vi "visualizrion.vi"() -> ()   [LabVIEW 2024]
uses:
  <vilib>/picture/3D Picture Control/Object/Create Object (name).vi
  <vilib>/Utility/file.llb/Read Delimited Spreadsheet (string).vi
  <vilib>/picture/3D Picture Control/Helpers/Set Light (no reference).vi
  <vilib>/picture/3D Picture Control/NI_3D Picture Control.lvlib
panel:
  out "Slide":u8(slide) scale=0.0..100.0
  in  "stop":bool
  out "3D Picture 2":refnum<vi>(3d-picture)
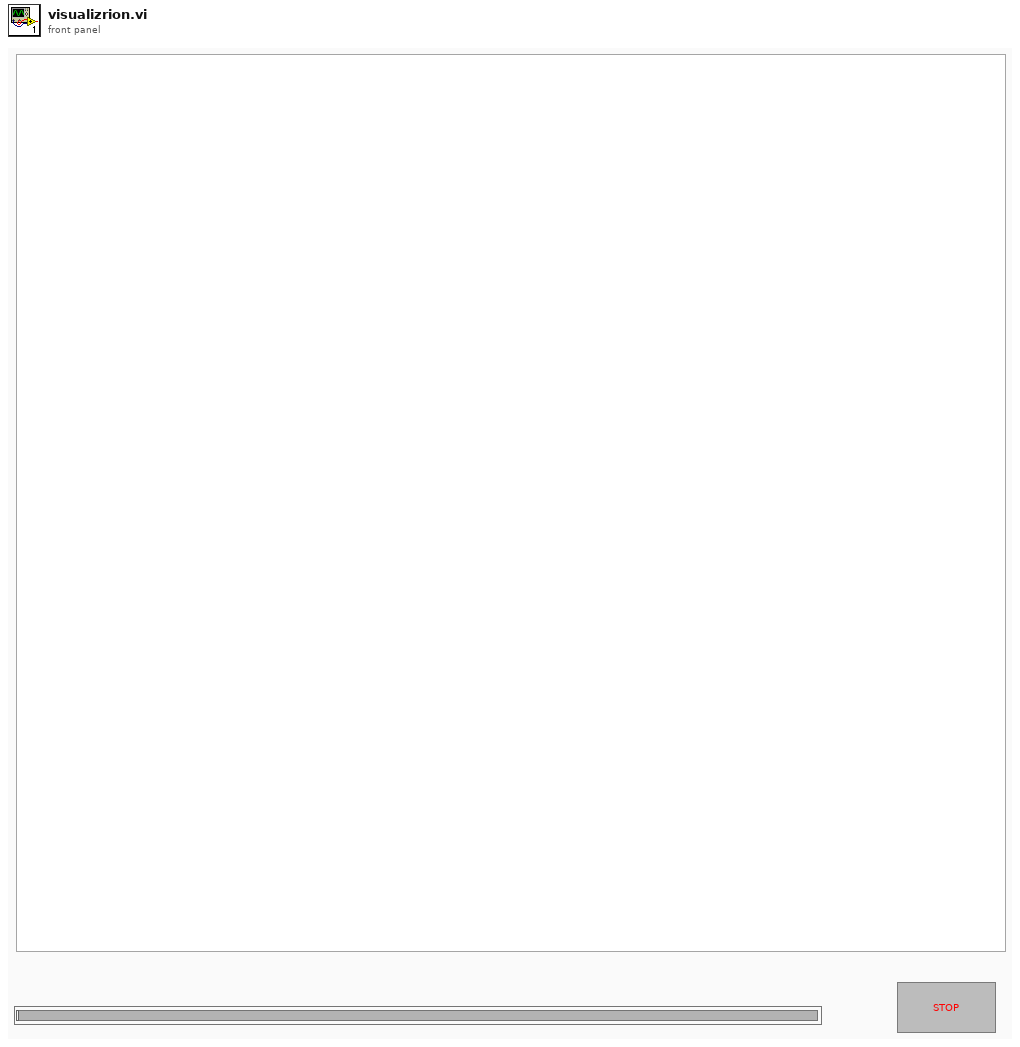
[diagram p1: front panel]
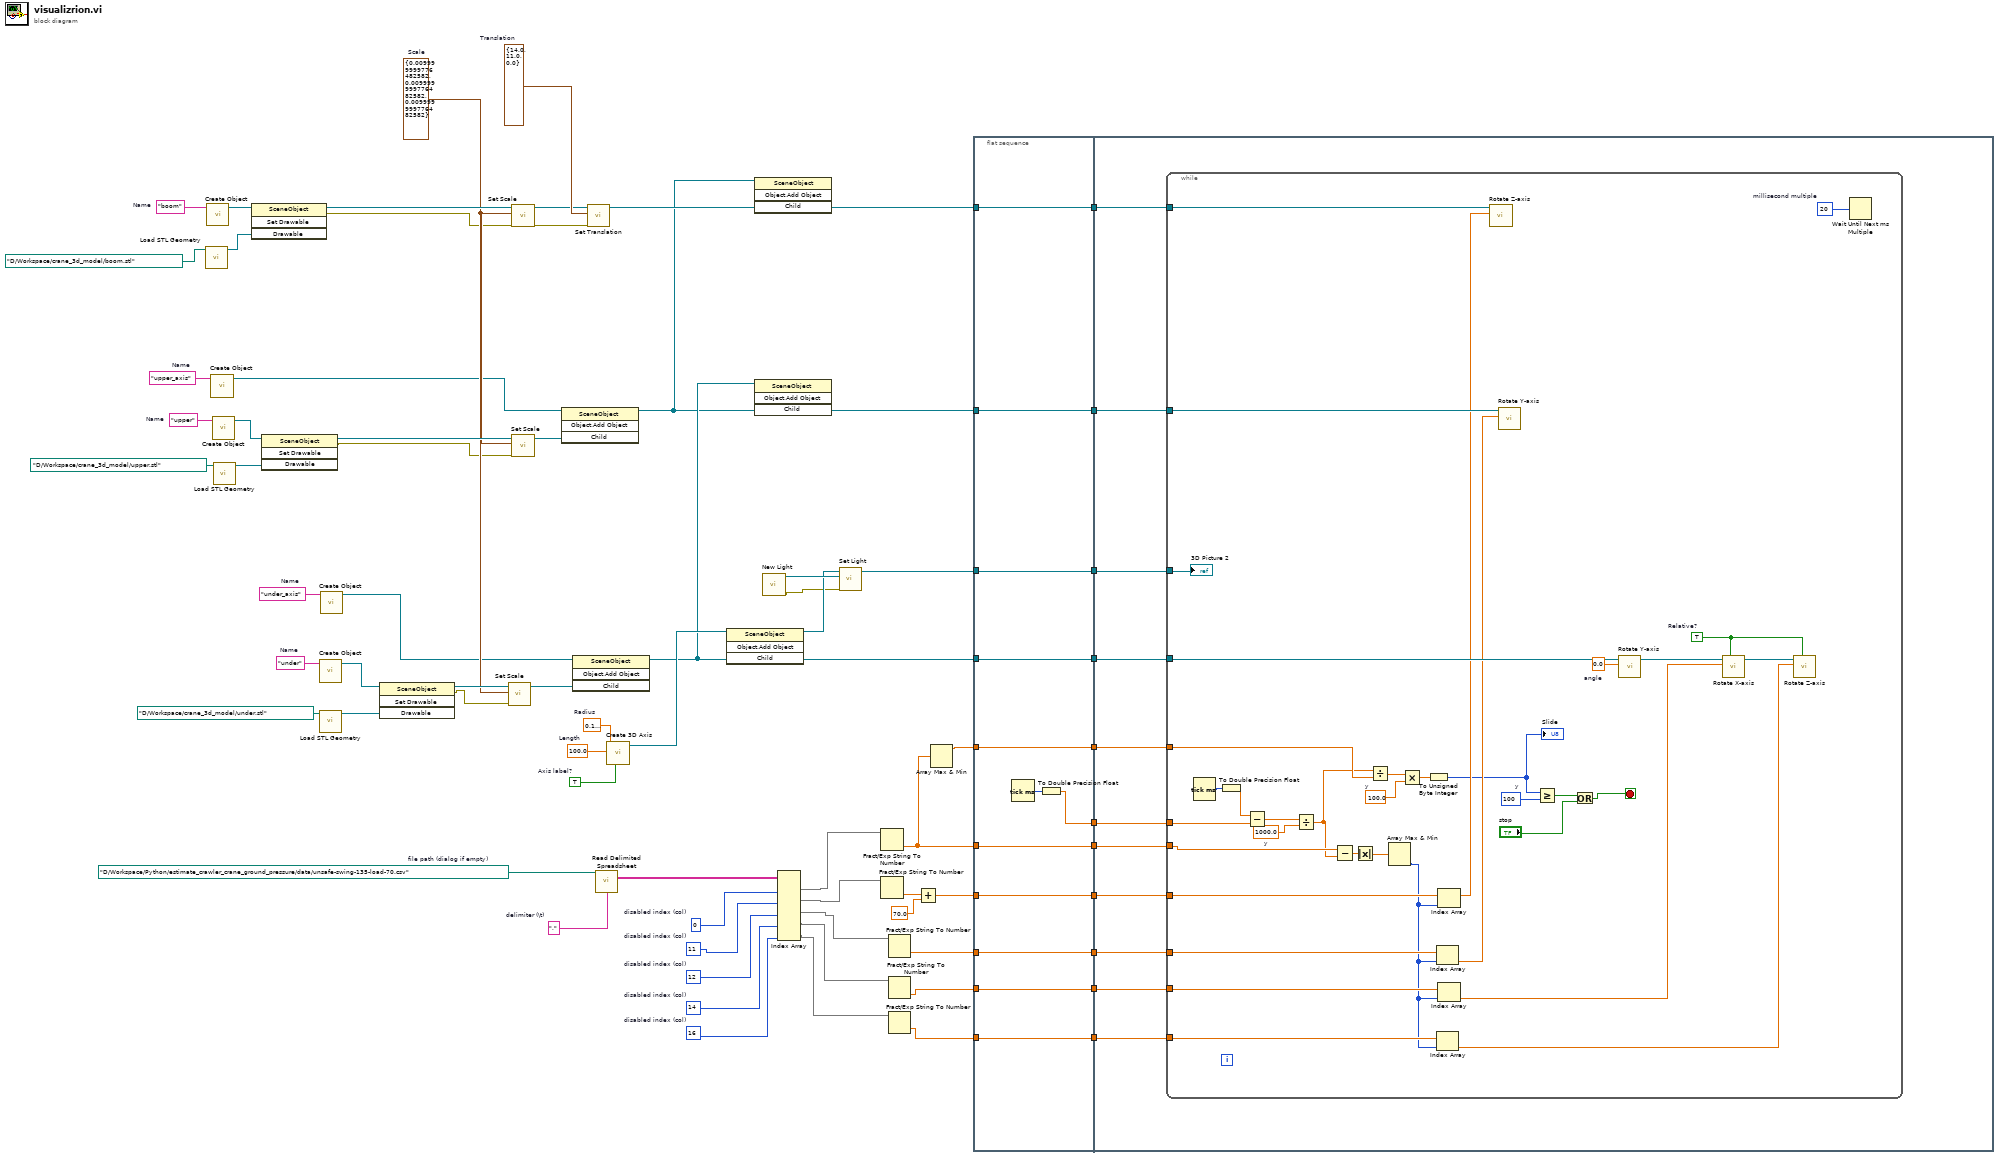
[diagram p0: block diagram]
diagram:
  w18 = 16  # disabled index (col)
  w19 = 14  # disabled index (col)
  w23 = 12  # disabled index (col)
  w28 = 11  # disabled index (col)
  w29 = 0  # disabled index (col)
  w31 = ","  # delimiter (\t)
  w32 = path "D:/Workspace/Python/estimate_crawler_crane_ground_pressure/data/unsafe-swing-135-load-70.csv"  # file path (dialog if empty)
  w43 = "upper_axis"  # Name
  w45 = "under_axis"  # Name
  w55 = cluster{"X":sgl, "Y":sgl, "Z":sgl} {"X"=14.0, "Y"=11.0, "Z"=0.0}  # Translation
  w53 = cluster{"X":sgl, "Y":sgl, "Z":sgl} {"X"=0.01, "Y"=0.01, "Z"=0.01}  # Scale
  w57 = "under"  # Name
  w62 = "upper"  # Name
  w66 = sgl 0.1  # Radius
  w69 = sgl 100.0  # Length
  w71 = TRUE  # Axis label?
  w72 = "boom"  # Name
  n1 = call <vilib>:"Load STL Geometry.vi"("Model File"=path "D:/Workspace/crane_3d_model/boom.stl") -> ("New Mesh Refnum"=w70:refnum<vi>)  [unwired: 9 in, 1 out]
  n2 = call-poly <vilib>:"Create Object.vi"("Name"=w72) -> ("Scene:New Object"=w73:refnum<vi>)  [unwired: 9 in, 1 out]
  n3 = call-poly <vilib>:"Create Object.vi"("Name"=w43) -> ("Scene:New Object"=w41:refnum<vi>)  [unwired: 9 in, 1 out]
  n4 = call-poly <vilib>:"Create Object.vi"("Name"=w62) -> ("Scene:New Object"=w64:refnum<vi>)  [unwired: 9 in, 1 out]
  n5 = call <vilib>:"Load STL Geometry.vi"("Model File"=path "D:/Workspace/crane_3d_model/upper.stl") -> ("New Mesh Refnum"=w61:refnum<vi>)  [unwired: 9 in, 1 out]
  n6 = invoke class="SceneObject" method="Set Drawable"(reference=w73, "Drawable"=w70) -> (reference out=w54:refnum<vi>, error out=w52:errorcluster)  [unwired: 2 in, 2 out]
  n7 = invoke class="SceneObject" method="Set Drawable"(reference=w64, "Drawable"=w61) -> (reference out=w63:refnum<vi>, error out=w39:errorcluster)  [unwired: 2 in, 2 out]
  n8 = call-poly <vilib>:"Create Object.vi"("Name"=w57) -> ("Scene:New Object"=w58:refnum<vi>)  [unwired: 9 in, 1 out]
  n9 = call <vilib>:"Load STL Geometry.vi"("Model File"=path "D:/Workspace/crane_3d_model/under.stl") -> ("New Mesh Refnum"=w56:refnum<vi>)  [unwired: 9 in, 1 out]
  n10 = call-poly <vilib>:"Create Object.vi"("Name"=w45) -> ("Scene:New Object"=w40:refnum<vi>)  [unwired: 9 in, 1 out]
  n11 = invoke class="SceneObject" method="Set Drawable"(reference=w58, "Drawable"=w56) -> (reference out=w60:refnum<vi>, error out=w49:errorcluster)  [unwired: 2 in, 2 out]
  n12 = call <vilib>:"Set Scale.vi"("error in (no error)"=w49, "Scale"=w53, "Scene Object"=w60) -> ("Scaled Object"=w44:refnum<vi>)  [unwired: 7 in, 1 out]
  n13 = call <vilib>:"Set Scale.vi"("error in (no error)"=w52, "Scale"=w53, "Scene Object"=w54) -> ("error out"=w50:errorcluster, "Scaled Object"=w51:refnum<vi>)  [unwired: 7 in]
  n14 = call <vilib>:"Set Scale.vi"("error in (no error)"=w39, "Scale"=w53, "Scene Object"=w63) -> ("Scaled Object"=w42:refnum<vi>)  [unwired: 7 in, 1 out]
  n15 = invoke class="SceneObject" method="Object.Add Object"(reference=w41, "Child"=w42) -> (reference out=w34:refnum<vi>)  [unwired: 2 in, 3 out]
  n16 = invoke class="SceneObject" method="Object.Add Object"(reference=w40, "Child"=w44) -> (reference out=w38:refnum<vi>)  [unwired: 2 in, 3 out]
  n17 = call <vilib>:"Set Translation.vi"("error in (no error)"=w50, "Translation"=w55, "Scene Object"=w51) -> ("Translated Object"=w35:refnum<vi>)  [unwired: 7 in, 1 out]
  n18 = call-poly <vilib>:"Read Delimited Spreadsheet.vi"("file path (dialog if empty)"=w32, "delimiter (\\t)"=w31) -> ("all rows"=w30:string[][])  [unwired: 8 in, 5 out]
  n19 = call <vilib>:"Create 3D Axis.vi"("Axis label?"=w71, "Radius"=w66, "Length"=w69) -> ("New Object Refnum"=w48:refnum<vi>)  [unwired: 7 in, 1 out]
  n20 = invoke class="SceneObject" method="Object.Add Object"(reference=w48, "Child"=w38) -> (reference out=w47:refnum<vi>, "Child"=w46:refnum<vi>)  [unwired: 2 in, 2 out]
  n21 = invoke class="SceneObject" method="Object.Add Object"(reference=w38, "Child"=w34) -> ("Child"=w37:refnum<vi>)  [unwired: 2 in, 3 out]
  n22 = invoke class="SceneObject" method="Object.Add Object"(reference=w34, "Child"=w35) -> ("Child"=w36:refnum<vi>)  [unwired: 2 in, 3 out]
  n23 = call <vilib>:"New Light.vi"() -> ("error out"=w33:errorcluster, "New Light Refnum"=w68:refnum<vi>)  [unwired: 10 in]
  n24 = Index Array(array=w30, index (col) #1=w29, index (col) #2=w28, index (col) #3=w23, index (col) #4=w19, index (col) #5=w18) -> (element #1=w20:string[], element #2=w21:string[], element #3=w22:string[], element #4=w17:string[], element #5=w16:string[])  [unwired: 5 in]
  n25 = call-poly <vilib>:"Set Light.vi"("error in (no error)"=w33, "Light Refnum In"=w68, "Scene Object In"=w47) -> ("Scene Object Out"=w67:refnum<vi>)  [unwired: 7 in, 1 out]
  n26 = Fract/Exp String To Number(string=w20) -> (number=w3:dbl[])  [unwired: 3 in, 1 out]
  n27 = Fract/Exp String To Number(string=w21) -> (number=w27:dbl[])  [unwired: 3 in, 1 out]
  n28 = Fract/Exp String To Number(string=w22) -> (number=w25:dbl[])  [unwired: 3 in, 1 out]
  n29 = Fract/Exp String To Number(string=w17) -> (number=w15:dbl[])  [unwired: 3 in, 1 out]
  n30 = Fract/Exp String To Number(string=w16) -> (number=w14:dbl[])  [unwired: 3 in, 1 out]
  n31 = Add(x=w27, y=70.0) -> (x+y=w24:dbl[])
  n32 = Array Max & Min(array=w3) -> (max value=w1:dbl)  [unwired: 3 out]
  n33 = flat-sequence {
    tunnel: w14 -> [w78]
    tunnel: w15 -> [w79]
    tunnel: w3 -> [w80]
    tunnel: w24 -> [w81]
    tunnel: w25 -> [w82]
    tunnel: w36 -> [w83]
    tunnel: w37 -> [w84]
    tunnel: w46 -> [w85]
    tunnel: w67 -> [w86]
    tunnel: [w86] -> w13
    tunnel: [w85] -> w12
    tunnel: [w84] -> w11
    tunnel: [w83] -> w10
    tunnel: [w82] -> w9
    tunnel: [w81] -> w8
    tunnel: [w80] -> w7
    tunnel: [w79] -> w6
    tunnel: [w78] -> w5
    tunnel: [w76] -> w4
    tunnel: [w75] -> w2
    tunnel: w1 -> [w75]
    tunnel: w13 -> [w97]
    tunnel: w12 -> [w96]
    tunnel: w11 -> [w95]
    tunnel: w10 -> [w94]
    tunnel: w9 -> [w93]
    tunnel: w8 -> [w92]
    tunnel: w7 -> [w91]
    tunnel: w6 -> [w90]
    tunnel: w5 -> [w89]
    tunnel: w4 -> [w88]
    tunnel: w2 -> [w87]
    frame #0 {
      n34 = Tick Count (ms)() -> (millisecond timer value=w77:u32)
      n35 = To Double Precision Float(number=w77) -> (double precision float=w76:dbl)
    }
    frame #1 {
      n36 = while {
        tunnel: w97 -> [w132]
        tunnel: w95 -> [w131]
        tunnel: w96 -> [w129]
        tunnel: w94 -> [w130]
        tunnel: w93 -> [w124]
        tunnel: w92 -> [w125]
        tunnel: w91 -> [w119]
        tunnel: w90 -> [w114]
        tunnel: w89 -> [w113]
        tunnel: w88 -> [w109]
        tunnel: w87 -> [w107]
        stop <- w98 stop-if-true
        w101 = u8 100  # y
        w104 = 100.0  # y
        w108 = 0.0  # angle
        w120 = 1000.0  # y
        w126 = TRUE  # Relative?
        w133 = u32 20  # millisecond multiple
        n37 = Tick Count (ms)() -> (millisecond timer value=w123:u32)
        n38 = To Double Precision Float(number=w123) -> (double precision float=w122:dbl)
        n39 = Subtract(x=w122, y=w109) -> (x-y=w121:dbl)
        n40 = Divide(x=w121, y=w120) -> (x/y=w106:dbl)
        n41 = Subtract(x=w119, y=w106) -> (x-y=w118:dbl[])
        n42 = Absolute Value(x=w118) -> (abs(x)=w117:dbl[])
        n43 = Divide(x=w106, y=w107) -> (x/y=w105:dbl)
        n44 = Array Max & Min(array=w117) -> (min index (indices)=w112:i32)  [unwired: 3 out]
        n45 = Multiply(x=w105, y=w104) -> (x*y=w103:dbl)
        n46 = To Unsigned Byte Integer(number=w103) -> (unsigned 8bit integer=w102:u8)
        "Slide" <- w102
        n47 = Index Array(array=w124, index=w112) -> (element=w115:dbl)
        n48 = Index Array(array=w113, index=w112) -> (element=w110:dbl)
        n49 = Index Array(array=w125, index=w112) -> (element=w116:dbl)
        n50 = Index Array(array=w114, index=w112) -> (element=w111:dbl)
        n51 = call <vilib>:"Rotate Z-axis.vi"("angle"=w116, "Scene Object In"=w130) -> ()  [unwired: 8 in, 2 out]
        n52 = call <vilib>:"Rotate Y-axis.vi"("angle"=w115, "Scene Object In"=w131) -> ()  [unwired: 8 in, 2 out]
        n53 = Greater Or Equal?(x=w102, y=w101) -> (x >= y?=w100:bool)
        n54 = Or(x=w100, y="stop") -> (x .or. y?=w98:bool)
        n55 = call <vilib>:"Rotate Y-axis.vi"("angle"=w108, "Scene Object In"=w129) -> ("Scene Object Out"=w128:refnum<vi>)  [unwired: 8 in, 1 out]
        n56 = call <vilib>:"Rotate X-axis.vi"("Relative?"=w126, "angle"=w111, "Scene Object In"=w128) -> ("Scene Object Out"=w127:refnum<vi>)  [unwired: 7 in, 1 out]
        n57 = call <vilib>:"Rotate Z-axis.vi"("Relative?"=w126, "angle"=w110, "Scene Object In"=w127) -> ()  [unwired: 7 in, 2 out]
        n58 = Wait Until Next ms Multiple(millisecond multiple=w133) -> ()  [unwired: 1 out]
        "3D Picture 2" <- w132
      }
    }
  }
